vi "CheckForErrorsInt.vi"(5 "Maximum":i32, 7 "Minimum":i32, 9 "Parameter Index":i32, 11 "Parameters":string[](array[string])) -> (0 "Error":errorcluster, 3 "Output":i32)   [LabVIEW 2019]
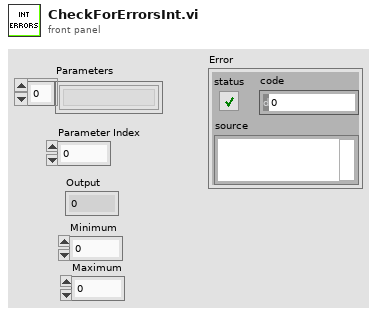
[diagram p1: front panel]
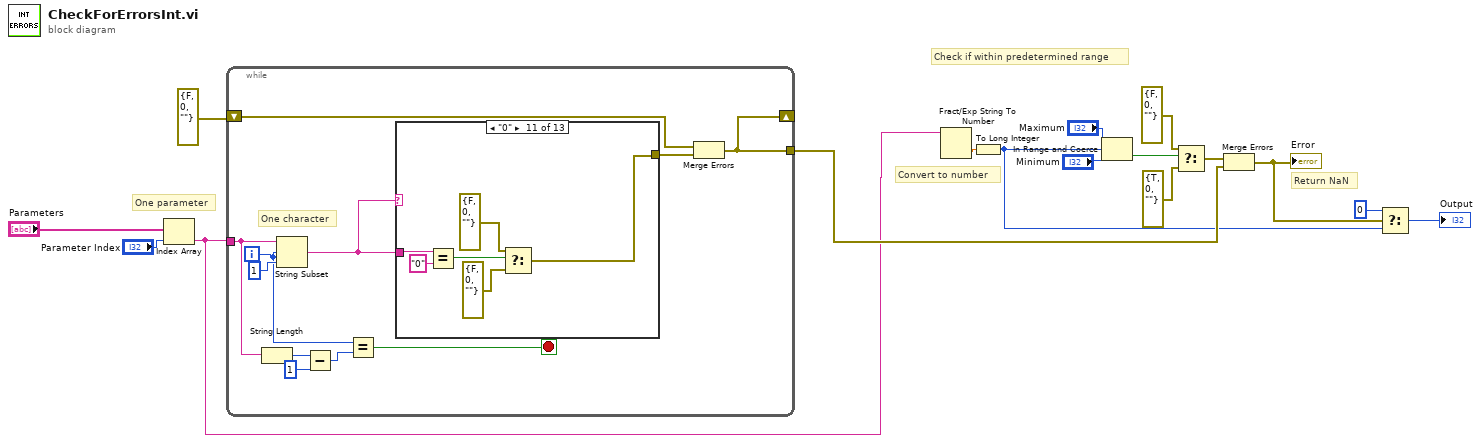
[diagram p0: block diagram]
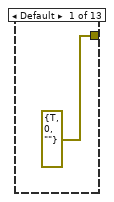
[diagram p2: hidden frame]
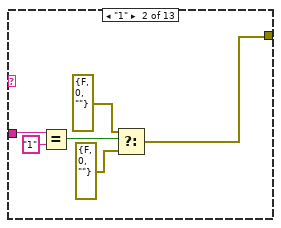
[diagram p3: hidden frame]
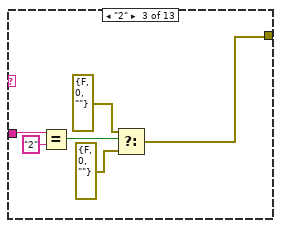
[diagram p4: hidden frame]
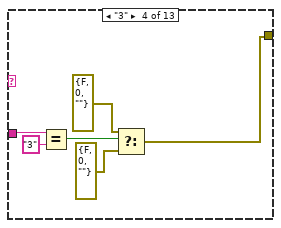
[diagram p5: hidden frame]
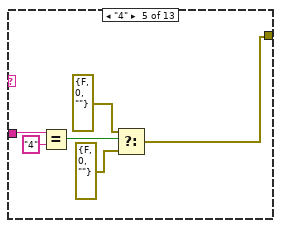
[diagram p6: hidden frame]
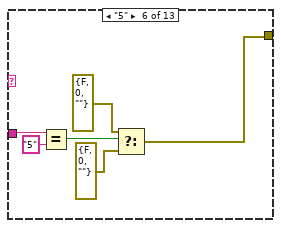
[diagram p7: hidden frame]
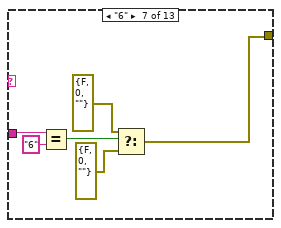
[diagram p8: hidden frame]
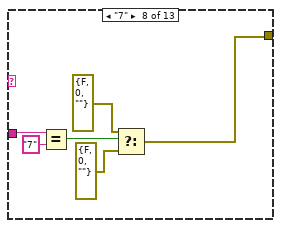
[diagram p9: hidden frame]
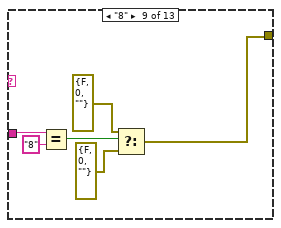
[diagram p10: hidden frame]
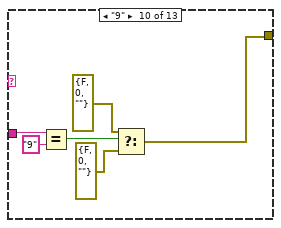
[diagram p11: hidden frame]
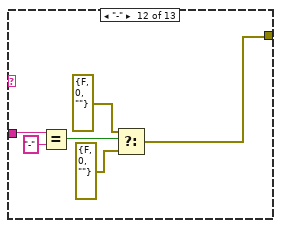
[diagram p12: hidden frame]
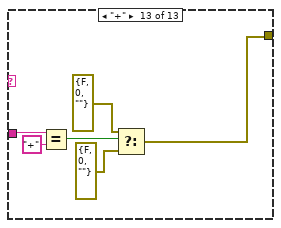
[diagram p13: hidden frame]
diagram:
  # "Convert to number"
  # "Return NaN"
  # "Check if within predetermined range"
  # "One parameter"
  n1 = Index Array(array="Parameters", index="Parameter Index") -> (element=w5:string)
  n2 = while {
    tunnel: w5 -> [w26]
    shift-right: [w17] -> _
    shift-left: errorcluster {"status"=FALSE, "code"=0, "source"=""} ("error constant") -> [w18]
    tunnel: [w17] -> w7
    i -> [w23]
    stop <- w25 stop-if-true
    # "One character"
    n3 = String Length(string=w26) -> (length=w22:i32)
    n4 = String Subset(string=w26, offset (0)=w23, length (rest)=1) -> (substring=w24:string)
    n5 = Subtract(x=w22, y=1) -> (x-y=w20:i32)
    n6 = Equal?(x=w23, y=w20) -> (x = y?=w25:bool)
    n7 = case shown="\"0\"" w24 {
      tunnel: w24 -> [_ w32 w38 w44 w50 w56 w62 w68 w74 w80 w86 w92 w98]
      tunnel: [errorcluster {"status"=TRUE, "code"=0, "source"=""} ("error constant") w29 w35 w41 w47 w53 w59 w65 w71 w77 w83 w89 w95] -> w19
      frame Default {
      }
      frame "1" {
        n8 = Equal?(x=w32, y="1") -> (x = y?=w33:bool)
        n9 = Select(t=errorcluster {"status"=FALSE, "code"=0, "source"=""} ("error constant"), s=w33, f=errorcluster {"status"=FALSE, "code"=0, "source"=""} ("error constant")) -> (s? t:f=w29:errorcluster)
      }
      frame "2" {
        n10 = Equal?(x=w38, y="2") -> (x = y?=w39:bool)
        n11 = Select(t=errorcluster {"status"=FALSE, "code"=0, "source"=""} ("error constant"), s=w39, f=errorcluster {"status"=FALSE, "code"=0, "source"=""} ("error constant")) -> (s? t:f=w35:errorcluster)
      }
      frame "3" {
        n12 = Equal?(x=w44, y="3") -> (x = y?=w45:bool)
        n13 = Select(t=errorcluster {"status"=FALSE, "code"=0, "source"=""} ("error constant"), s=w45, f=errorcluster {"status"=FALSE, "code"=0, "source"=""} ("error constant")) -> (s? t:f=w41:errorcluster)
      }
      frame "4" {
        n14 = Equal?(x=w50, y="4") -> (x = y?=w51:bool)
        n15 = Select(t=errorcluster {"status"=FALSE, "code"=0, "source"=""} ("error constant"), s=w51, f=errorcluster {"status"=FALSE, "code"=0, "source"=""} ("error constant")) -> (s? t:f=w47:errorcluster)
      }
      frame "5" {
        n16 = Equal?(x=w56, y="5") -> (x = y?=w57:bool)
        n17 = Select(t=errorcluster {"status"=FALSE, "code"=0, "source"=""} ("error constant"), s=w57, f=errorcluster {"status"=FALSE, "code"=0, "source"=""} ("error constant")) -> (s? t:f=w53:errorcluster)
      }
      frame "6" {
        n18 = Equal?(x=w62, y="6") -> (x = y?=w63:bool)
        n19 = Select(t=errorcluster {"status"=FALSE, "code"=0, "source"=""} ("error constant"), s=w63, f=errorcluster {"status"=FALSE, "code"=0, "source"=""} ("error constant")) -> (s? t:f=w59:errorcluster)
      }
      frame "7" {
        n20 = Equal?(x=w68, y="7") -> (x = y?=w69:bool)
        n21 = Select(t=errorcluster {"status"=FALSE, "code"=0, "source"=""} ("error constant"), s=w69, f=errorcluster {"status"=FALSE, "code"=0, "source"=""} ("error constant")) -> (s? t:f=w65:errorcluster)
      }
      frame "8" {
        n22 = Equal?(x=w74, y="8") -> (x = y?=w75:bool)
        n23 = Select(t=errorcluster {"status"=FALSE, "code"=0, "source"=""} ("error constant"), s=w75, f=errorcluster {"status"=FALSE, "code"=0, "source"=""} ("error constant")) -> (s? t:f=w71:errorcluster)
      }
      frame "9" {
        n24 = Equal?(x=w80, y="9") -> (x = y?=w81:bool)
        n25 = Select(t=errorcluster {"status"=FALSE, "code"=0, "source"=""} ("error constant"), s=w81, f=errorcluster {"status"=FALSE, "code"=0, "source"=""} ("error constant")) -> (s? t:f=w77:errorcluster)
      }
      frame "0" {
        n26 = Equal?(x=w86, y="0") -> (x = y?=w87:bool)
        n27 = Select(t=errorcluster {"status"=FALSE, "code"=0, "source"=""} ("error constant"), s=w87, f=errorcluster {"status"=FALSE, "code"=0, "source"=""} ("error constant")) -> (s? t:f=w83:errorcluster)
      }
      frame "-" {
        n28 = Equal?(x=w92, y="-") -> (x = y?=w93:bool)
        n29 = Select(t=errorcluster {"status"=FALSE, "code"=0, "source"=""} ("error constant"), s=w93, f=errorcluster {"status"=FALSE, "code"=0, "source"=""} ("error constant")) -> (s? t:f=w89:errorcluster)
      }
      frame "+" {
        n30 = Equal?(x=w98, y="+") -> (x = y?=w99:bool)
        n31 = Select(t=errorcluster {"status"=FALSE, "code"=0, "source"=""} ("error constant"), s=w99, f=errorcluster {"status"=FALSE, "code"=0, "source"=""} ("error constant")) -> (s? t:f=w95:errorcluster)
      }
    }
    n32 = Merge Errors(w18, w19) -> (w17:errorcluster)
  }
  n33 = Fract/Exp String To Number(string=w5) -> (number=w2:dbl)  [unwired: 3 in, 1 out]
  n34 = To Long Integer(number=w2) -> (32bit integer=w1:i32)
  n35 = In Range and Coerce(upper limit="Maximum", x=w1, lower limit="Minimum") -> (In Range?=w11:bool)  [unwired: 1 out]
  n36 = Select(t=errorcluster {"status"=FALSE, "code"=0, "source"=""} ("error constant"), s=w11, f=errorcluster {"status"=TRUE, "code"=0, "source"=""} ("error constant")) -> (s? t:f=w8:errorcluster)
  n37 = Merge Errors(w8, w7) -> (w4:errorcluster)
  "Error" <- w4
  n38 = Select(t=0, s=w4, f=w1) -> (s? t:f=→"Output":i32)
